vi "Copy.vi"(0 "Case Structure in":refnum<class "Case Structure.lvclass">, 1 "Linked List Ref":refnum<data-value>, 2 "New Parent ID":string, 5 "Test ID":string, 7 "Insertion Index":i32=-1, 9 "Move?":bool, 11 "error in (no error)":errorcluster, 12 "New ID":string, 13 "Data IDs":variant) -> (3 "Linked List Ref out":refnum<data-value>, 6 "Linked List ID out":string, 14 "Data IDs out":variant, 15 "error out":errorcluster)   [LabVIEW 2017, in "Custom Type Test Executive.lvlib" / "Case Structure.lvclass"]
uses:
  <vilib>/gpm_packages/@cs/test-executive/Source/Custom Type Test Executive/Case Structure/Case Structure.lvclass
  <vilib>/gpm_packages/@cs/linked-list/Source/Linked List/ILinkedList/ILinked List.lvclass
  <vilib>/gpm_packages/@cs/data-type-serializer/source/String/String.lvclass/String.ctl
  <vilib>/gpm_packages/@cs/test-executive/Source/Test Executive/Executioner/Executioner.lvclass
  <vilib>/gpm_packages/@cs/data-type-serializer/source/String 1D/String 1D.lvclass/String 1D.ctl
  2c72c30c-231e-45ac-9cb8-eb055cf78a22.vi
  77bc07aa-e694-4b7b-8317-4810ec6c4467.vi
  21b2d93f-008a-42cf-b2d5-219c00c76e28.vi
  9dc23424-4fbb-414d-85ae-ea94ea9941f2.vi
  f13c266f-8cc9-455f-9976-00cb2d1b3653.vi
  c0a370ed-d996-43d3-98e7-38dfea424476.vi
  733ee169-be2d-4464-82bc-6d450e61d95e.vi
  81dc1bac-c7a2-4768-8037-82e71031ad61.vi
  <vilib>/gpm_packages/@cs/data-type-serializer/source/String 1D/String 1D.lvclass
  C:/Program Files/National Instruments/LabVIEW 2017/vi.lib/gpm_packages/@cs/data-type-serializer/source/Data Type/Data Type.lvclass
  <vilib>/gpm_packages/@cs/data-type-serializer/source/String/String.lvclass
  <vilib>/gpm_packages/@cs/linked-list/Source/Linked List/Linked List Ref/Linked List Ref.lvclass
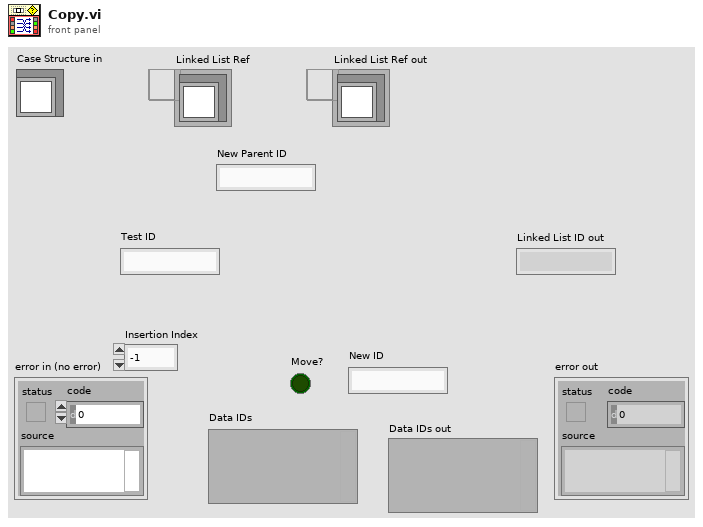
[diagram p1: front panel]
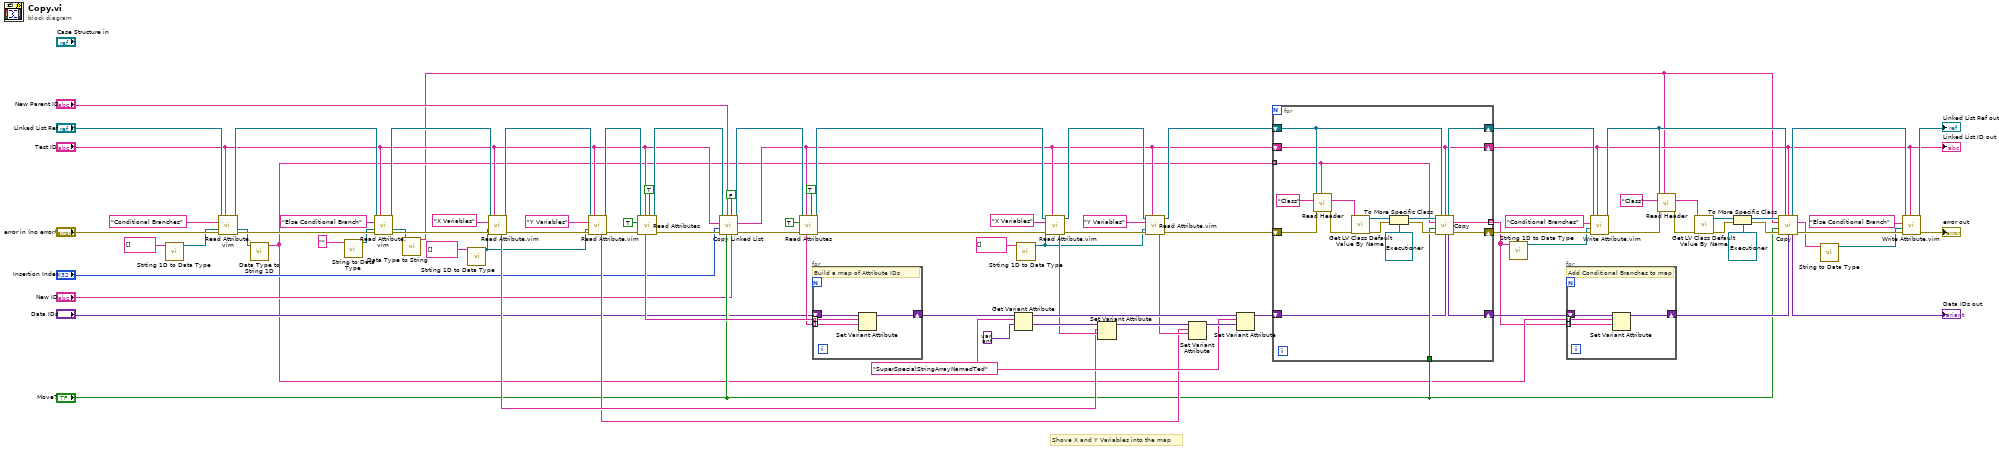
[diagram p0: block diagram]
diagram:
  w48 = "SuperSpecialStringArrayNamedTed" ("name")
  # "Shove X and Y Variables into the map"
  n1 = call <vilib>:"Strting 1D to Data Type.vi"("String 1D"=string[] []) -> ("Boolean out"=w15:refnum<class "String 1D.lvclass">)  [unwired: 9 in, 1 out]
  n2 = call "Read Attribute.vim"("Linked List Ref"="Linked List Ref", "Linked List ID"="Test ID", "Attribute Name"="Conditional Branches", "Type"=w15, "error in (no error)"="error in (no error)") -> ("Linked List Ref out"=w86:refnum<data-value>, "Attribute"=w14:refnum<class "String 1D.lvclass">, "error out"=w87:errorcluster)  [unwired: 5 in, 3 out]
  n3 = call <vilib>:"Data Type to String 1D.vi"("Data Type"=w14) -> ("String 1D out"=w13:string[])  [unwired: 9 in, 1 out]
  n4 = call <vilib>:"String to Data Type.vi"("String"="") -> ("Boolean out"=w11:refnum<class "String.lvclass">)  [unwired: 9 in, 1 out]
  n5 = call "Read Attribute.vim"("Linked List Ref"=w86, "Linked List ID"="Test ID", "Attribute Name"="Else Conditional Branch", "Type"=w11, "error in (no error)"=w87) -> ("Linked List Ref out"=w56:refnum<data-value>, "Attribute"=w10:refnum<class "String.lvclass">, "error out"=w58:errorcluster)  [unwired: 5 in, 3 out]
  n6 = call <vilib>:"Data Type to String.vi"("Data Type"=w10) -> ("String out"=w9:string)  [unwired: 9 in, 1 out]
  n7 = call <vilib>:"Strting 1D to Data Type.vi"("String 1D"=string[] []) -> ("Boolean out"=w7:refnum<class "String 1D.lvclass">)  [unwired: 9 in, 1 out]
  n8 = call "Read Attribute.vim"("Linked List Ref"=w56, "Linked List ID"="Test ID", "Attribute Name"="X Variables", "Type"=w7, "error in (no error)"=w58) -> ("Linked List Ref out"=w55:refnum<data-value>, "Data ID"=w32:string, "error out"=w59:errorcluster)  [unwired: 5 in, 3 out]
  n9 = call "Read Attribute.vim"("Linked List Ref"=w55, "Linked List ID"="Test ID", "Attribute Name"="Y Variables", "Type"=w7, "error in (no error)"=w59) -> ("Linked List Ref out"=w54:refnum<data-value>, "Data ID"=w31:string, "error out"=w57:errorcluster)  [unwired: 5 in, 3 out]
  n10 = call <vilib>:"Read Attributes.vi"("Flatten Pointer?"=TRUE, "Linked List ID"="Test ID", "error in (no error)"=w57, "Include Private?"=TRUE, "Linked List Ref"=w54) -> ("error out"=w63:errorcluster, "Linked List Ref out"=w62:refnum<data-value>, "Data IDs"=w51:string[])  [unwired: 1 in, 3 out]
  n11 = call <vilib>:"Copy Linked List.vi"("New Linked List ID"="New ID", "Recursive? (T)"=FALSE, "Move?"="Move?", "New Parent Linked List ID"="New Parent ID", "error in (no error)"=w63, "Insertion Index"="Insertion Index", "Linked List ID"="Test ID", "Linked List Ref"=w62) -> ("error out"=w67:errorcluster, "Linked List ID out"=w33:string, "Linked List Ref out"=w66:refnum<data-value>)  [unwired: 1 out]
  n12 = call <vilib>:"Read Attributes.vi"("Flatten Pointer?"=TRUE, "Linked List ID"=w33, "error in (no error)"=w67, "Include Private?"=TRUE, "Linked List Ref"=w66) -> ("error out"=w40:errorcluster, "Linked List Ref out"=w36:refnum<data-value>, "Data IDs"=w50:string[])  [unwired: 1 in, 3 out]
  n13 = for {
    tunnel: w51 -> [w93] mode=indexing
    tunnel: w50 -> [w92] mode=indexing
    shift-right: [w91] -> w30
    shift-left: "Data IDs" -> [w94]
    # "Build a map of Attribute IDs"
    n14 = Set Variant Attribute(Variant=w94, name=w93, value=w92) -> (Variant out=w91:variant)  [unwired: 1 in, 2 out]
  }
  n15 = Get Variant Attribute(Variant=w30, name=w48, default value (empty Variant)=variant ("default value (empty variant)")) -> (duplicate Variant=w47:variant, value=w45:variant)  [unwired: 1 in, 2 out]
  n16 = call <vilib>:"Strting 1D to Data Type.vi"("String 1D"=string[] []) -> ("Boolean out"=w5:refnum<class "String 1D.lvclass">)  [unwired: 9 in, 1 out]
  n17 = call "Read Attribute.vim"("Linked List Ref"=w36, "Linked List ID"=w33, "Attribute Name"="X Variables", "Type"=w5, "error in (no error)"=w40) -> ("Linked List Ref out"=w35:refnum<data-value>, "Data ID"=w38:string, "error out"=w41:errorcluster)  [unwired: 5 in, 3 out]
  n18 = Set Variant Attribute(Variant=w45, name=w32, value=w38) -> (Variant out=w46:variant)  [unwired: 1 in, 2 out]
  n19 = call "Read Attribute.vim"("Linked List Ref"=w35, "Linked List ID"=w33, "Attribute Name"="Y Variables", "Type"=w5, "error in (no error)"=w41) -> ("Linked List Ref out"=w34:refnum<data-value>, "Data ID"=w37:string, "error out"=w39:errorcluster)  [unwired: 5 in, 3 out]
  n20 = Set Variant Attribute(Variant=w46, name=w31, value=w37) -> (Variant out=w49:variant)  [unwired: 1 in, 2 out]
  n21 = Set Variant Attribute(Variant=w47, name=w48, value=w49) -> (Variant out=w29:variant)  [unwired: 1 in, 2 out]
  n22 = for {
    tunnel: "Move?" -> [w100]
    tunnel: w13 -> [w99] mode=indexing
    shift-right: [w102] -> w85
    shift-left: w39 -> [w104]
    shift-right: [w101] -> w83
    shift-left: w34 -> [w103]
    shift-right: [w98] -> w17
    shift-left: w33 -> [w98]
    tunnel: [w97] -> w3 mode=indexing
    shift-right: [w95] -> w61
    shift-left: w29 -> [w96]
    n23 = call <vilib>:"Read Header.vi"("Linked List ID"=w99, "error in (no error)"=w104, "Header Name"="Class", "Linked List Ref"=w103) -> ("error out"=w109:errorcluster, "Header Value"=w111:string)  [unwired: 4 in, 2 out]
    n24 = call <vilib>:"Get LV Class Default Value By Name.vi"("error in (no error)"=w109, "class name"=w111) -> ("error out"=w108:errorcluster, "object"=w110:refnum<class>)  [unwired: 8 in]
    n25 = To More Specific Class(target class=refnum<class "Executioner.lvclass"> refnum ("Test Executive.lvlib:Executioner.lvclass"), reference=w110, error in=w108) -> (specific class reference=w105:refnum<class "Executioner.lvclass">, error out=w106:errorcluster)
    n26 = call-dynamic "Copy.vi"("Executioner in"=w105, "Linked List Ref"=w103, "New Parent ID"=w98, "Test ID"=w99, "Move?"=w100, "error in (no error)"=w106, "Data IDs"=w96) -> ("Linked List Ref out"=w101:refnum<data-value>, "Linked List ID out"=w97:string, "Data IDs out"=w95:variant, "error out"=w102:errorcluster)  [unwired: 5 in]
  }
  "Linked List ID out" <- w17
  n27 = call <vilib>:"Strting 1D to Data Type.vi"("String 1D"=w3) -> ("Boolean out"=w4:refnum<class "String 1D.lvclass">)  [unwired: 9 in, 1 out]
  n28 = for {
    tunnel: w13 -> [w115] mode=indexing
    tunnel: w3 -> [w114] mode=indexing
    shift-right: [w113] -> w60
    shift-left: w61 -> [w116]
    # "Add Conditional Branches to map"
    n29 = Set Variant Attribute(Variant=w116, name=w115, value=w114) -> (Variant out=w113:variant)  [unwired: 1 in, 2 out]
  }
  n30 = call "Write Attribute.vim"("Linked List ID"=w17, "error in (no error)"=w85, "Attribute"=w4, "Attribute Name"="Conditional Branches", "Linked List Ref"=w83) -> ("error out"=w70:errorcluster, "Linked List Ref out"=w71:refnum<data-value>)  [unwired: 3 in, 2 out]
  n31 = call <vilib>:"Read Header.vi"("Linked List ID"=w9, "error in (no error)"=w70, "Header Name"="Class", "Linked List Ref"=w71) -> ("error out"=w75:errorcluster, "Header Value"=w73:string)  [unwired: 4 in, 2 out]
  n32 = call <vilib>:"Get LV Class Default Value By Name.vi"("error in (no error)"=w75, "class name"=w73) -> ("error out"=w76:errorcluster, "object"=w74:refnum<class>)  [unwired: 8 in]
  n33 = To More Specific Class(target class=refnum<class "Executioner.lvclass"> refnum ("Test Executive.lvlib:Executioner.lvclass"), reference=w74, error in=w76) -> (specific class reference=w79:refnum<class "Executioner.lvclass">, error out=w78:errorcluster)
  n34 = call-dynamic "Copy.vi"("Executioner in"=w79, "Linked List Ref"=w71, "New Parent ID"=w17, "Test ID"=w9, "Move?"="Move?", "error in (no error)"=w78, "Data IDs"=w60) -> ("Linked List Ref out"=w82:refnum<data-value>, "Linked List ID out"=w2:string, "Data IDs out"=→"Data IDs out":variant, "error out"=w80:errorcluster)  [unwired: 5 in]
  n35 = call <vilib>:"String to Data Type.vi"("String"=w2) -> ("Boolean out"=w1:refnum<class "String.lvclass">)  [unwired: 9 in, 1 out]
  n36 = call "Write Attribute.vim"("Linked List ID"=w17, "error in (no error)"=w80, "Attribute"=w1, "Attribute Name"="Else Conditional Branch", "Linked List Ref"=w82) -> ("error out"=→"error out":errorcluster, "Linked List Ref out"=→"Linked List Ref out":refnum<data-value>)  [unwired: 3 in, 2 out]
